vi "ReadVSChEventOutgoing.vi"(7 "EventFRActive?":bool, 8 "error in (no error)":errorcluster, 10 "EventFrames list":T1[](array[typedef]) {"Channel Data Ref" format="%.0x"}, 11 "Refnum in":refnum<k21>[](array[refnum])) -> (0 "error out":errorcluster, 2 "EventFrames list Out":T1[](array[typedef]) {"Channel Data Ref" format="%.0x"}, 3 "Refnum out":refnum<k21>[](array[refnum]))   [LabVIEW 2020, in "FlexRay Custom Device Engine.lvlib"]
uses:
  FlexRay Custom Device Engine.lvlib
  Shared/FREventInfo.ctl
  <vilib>/NI VeriStand/Custom Device API/Data Reference.ctl
  <vilib>/NI VeriStand/Custom Device API/Global Data Refs.vi
  <vilib>/xnet/xnet.llb/XNET Write (Signal Single-point).vi
  <vilib>/NI VeriStand/Custom Device API/Custom Device API.lvlib
  Shared/FlexRay Custom Device Shared.lvlib
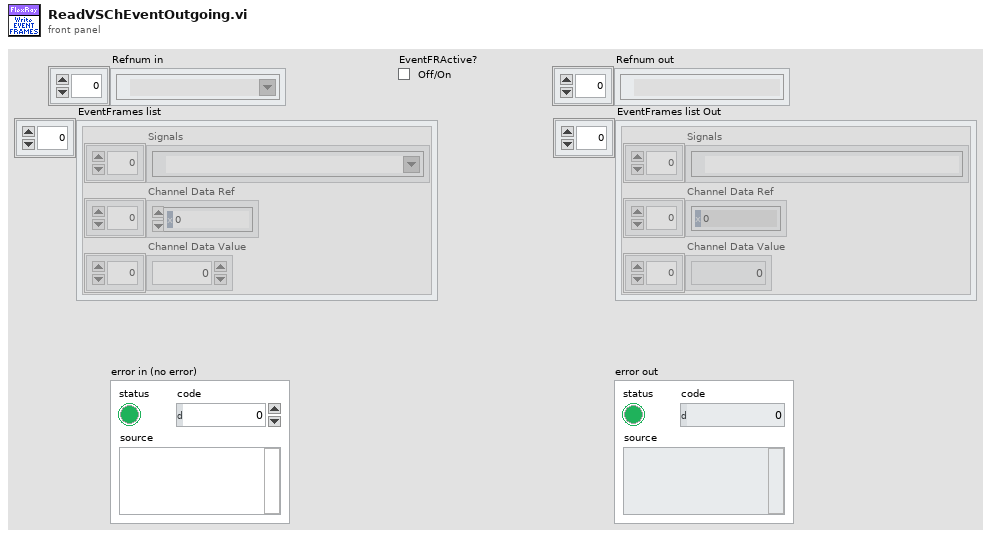
[diagram p1: front panel]
types:
  T1 = typedef "FlexRay Custom Device Shared.lvlib/FREventInfo.ctl" = cluster{"Signals":refnum<k21>[], "Channel Data Ref":T2[], "Channel Data Value":dbl[]}
  T2 = typedef "Custom Device API.lvlib/Data Reference.ctl" = i32
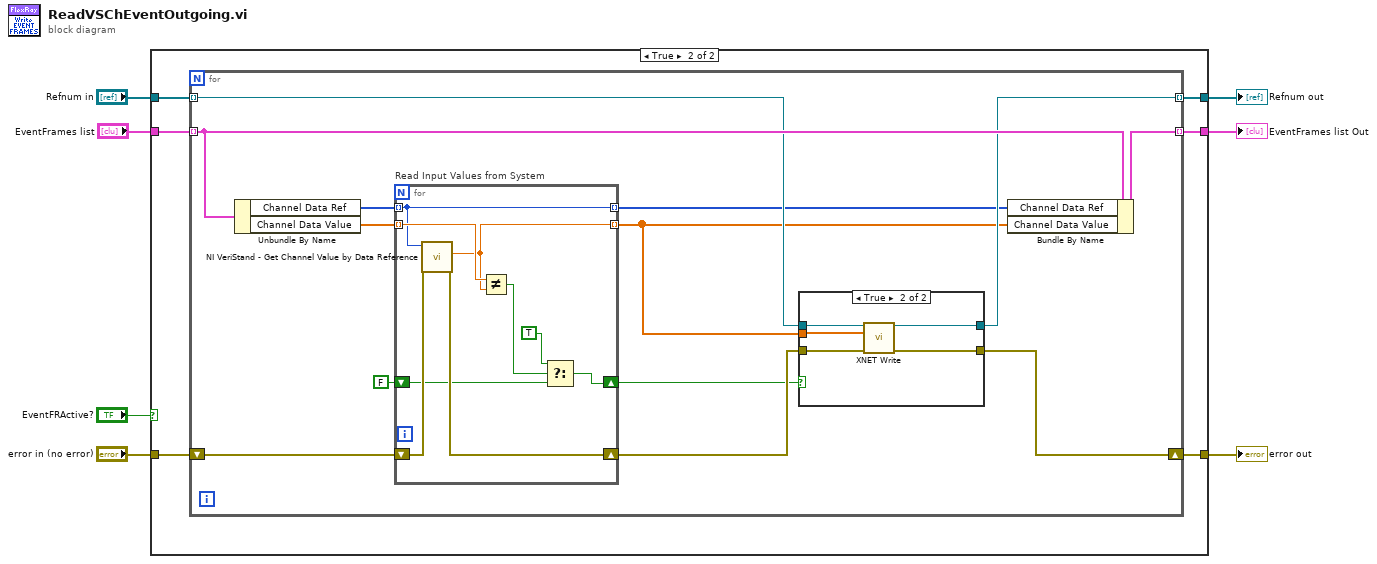
[diagram p0: block diagram]
diagram:
  n1 = case shown="True" "EventFRActive?" {
    tunnel: [w9 w13] -> w7
    tunnel: [w10 w16] -> w6
    tunnel: "error in (no error)" -> [w10 w15]
    tunnel: "Refnum in" -> [w9 w14]
    tunnel: "EventFrames list" -> [w8 w12]
    tunnel: [w8 w11] -> w1
    frame False {
    }
    frame True {
      n2 = for {
        shift-right: [w25] -> w16
        shift-left: w15 -> [w29]
        tunnel: w14 -> [w24] mode=indexing
        tunnel: [w26] -> w13 mode=indexing
        tunnel: w12 -> [w28] mode=indexing
        tunnel: [w27] -> w11 mode=indexing
        n3 = Unbundle By Name(w28) -> ("Channel Data Ref"=w23:T2[], "Channel Data Value"=w22:dbl[])
        n4 = for "Read Input Values from System" {
          shift-right: [w44] -> w20
          shift-left: w29 -> [w45]
          tunnel: w23 -> [w42] mode=indexing
          tunnel: w22 -> [w43] mode=indexing
          tunnel: [w42] -> w21 mode=indexing
          shift-right: [w38] -> w18
          shift-left: FALSE -> [w40]
          tunnel: [w37] -> w17 mode=indexing
          n5 = call <vilib>:"NI VeriStand - Get Channel Value by Data Reference.vi"("error in (no error)"=w45, "Data Reference in"=w42) -> ("error out"=w44:errorcluster, "Value"=w37:dbl)  [unwired: 8 out]
          n6 = Not Equal?(x=w43, y=w37) -> (x != y?=w41:bool)
          n7 = Select(t=TRUE, s=w41, f=w40) -> (s? t:f=w38:bool)
        }
        n8 = case shown="True" w18 {
          tunnel: w20 -> [w31 w36]
          tunnel: [w30 w35] -> w26
          tunnel: [w31 w34] -> w25
          tunnel: w24 -> [w30 w33]
          tunnel: w17 -> [_ w32]
          frame False {
          }
          frame True {
            n9 = call-poly <vilib>:"XNET Write.vi"("session in"=w33, "data"=w32, "error in (no error)"=w36) -> ("session out"=w35:refnum<k21>, "error out"=w34:errorcluster)  [unwired: 11 in]
          }
        }
        n10 = Bundle By Name(cluster=w28, "Channel Data Ref"=w21, "Channel Data Value"=w17) -> (w27:T1)
      }
    }
  }
  "Refnum out" <- w7
  "error out" <- w6
  "EventFrames list Out" <- w1
